vi "FPGA_read_laser_array_for_FPGA.vi"(2 "Laser lines array":dbl[][](array[numeric]), 3 "Illumination source":bool) -> (0 "Laser power":sgl[](array[numeric]), 1 "Laser lines":i32[](array[numeric]))   [LabVIEW 2015]
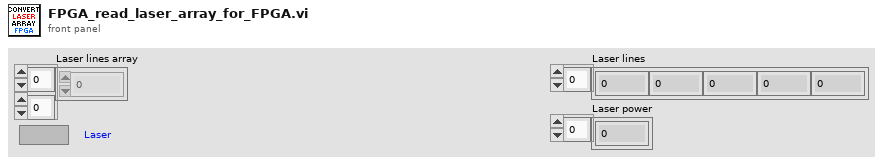
[diagram p1: front panel]
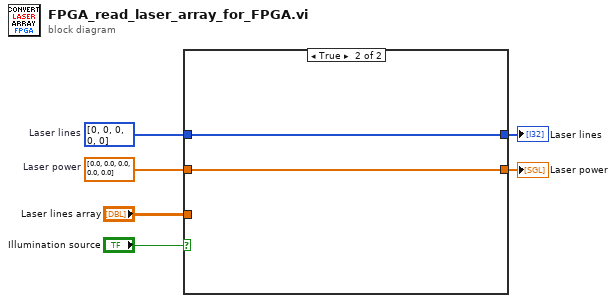
[diagram p0: block diagram]
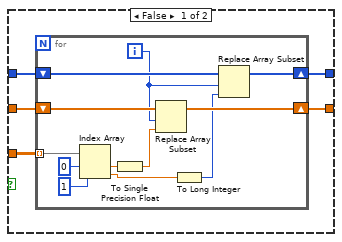
[diagram p2: hidden frame]
diagram:
  w5 = sgl[] [0.0, 0.0, 0.0, 0.0, 0.0]  # Laser power
  w6 = i32[] [0, 0, 0, 0, 0]  # Laser lines
  n1 = case shown="True" "Illumination source" {
    tunnel: w6 -> [w11 w25]
    tunnel: w5 -> [w10 w24]
    tunnel: "Laser lines array" -> [w9 _]
    tunnel: [w8 w25] -> w3
    tunnel: [w7 w24] -> w2
    frame False {
      n2 = for {
        shift-right: [w16] -> w8
        shift-left: w11 -> [w17]
        shift-right: [w20] -> w7
        shift-left: w10 -> [w21]
        tunnel: w9 -> [w23] mode=indexing
        i -> [w15]
        n3 = Index Array(array=w23, index #1=0 ("index"), index #2=1 ("index")) -> (element #1=w19:dbl, element #2=w13:dbl)
        n4 = To Single Precision Float(number=w19) -> (single precision float=w18:sgl)
        n5 = Replace Array Subset(array=w21, new element=w18, index=w15) -> (w20:sgl[])
        n6 = To Long Integer(number=w13) -> (32bit integer=w12:i32)
        n7 = Replace Array Subset(array=w17, new element=w12, index=w15) -> (w16:i32[])
      }
    }
    frame True {
    }
  }
  "Laser lines" <- w3
  "Laser power" <- w2
